vi "Write Waveform Type.vi"(8 "error in":errorcluster, 10 "Waveform Type":T1, 11 "Function Generator in":refnum<class "Function Generator.lvclass">) -> (0 "error out":errorcluster, 3 "Function Generator out":refnum<class "Function Generator.lvclass">)   [LabVIEW 2018, in "Function Generator.lvlib" / "Function Generator.lvclass"]
uses:
  Function Generator.lvclass
  Custom Controls/Waveform Type.ctl
  Function Generator.lvclass/Function Generator.ctl
  Function Generator.lvlib
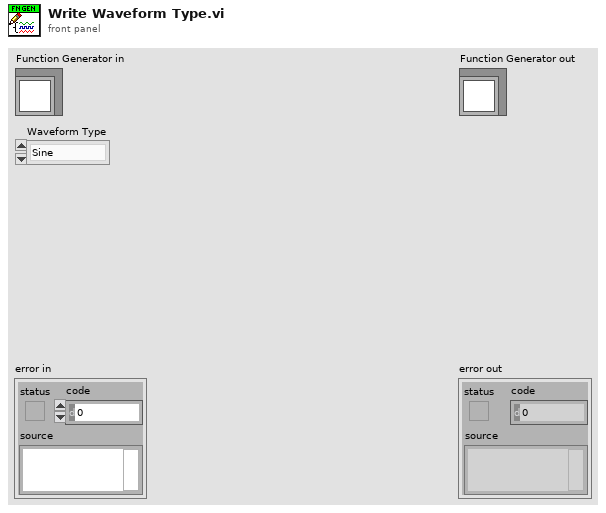
[diagram p1: front panel]
types:
  T1 = typedef "Function Generator.lvlib/Waveform Type.ctl" = enum16{"Sine", "Square", "Triangle", "Sawtooth", "DC"}
  T2 = typedef "Function Generator.lvlib/Channel Settings.ctl" = cluster{"Waveform Type":T1, "Amplitude Pk-Pk(V)":dbl, "Duty Cycle (%)":dbl, "Frequency (Hz)":dbl, "DC offset":dbl, "Output":bool}
  T3 = typedef "Function Generator.lvlib/Channel.ctl" = enum16{"Channel 1", "Channel 2", "Channel 3", "Channel 4"}
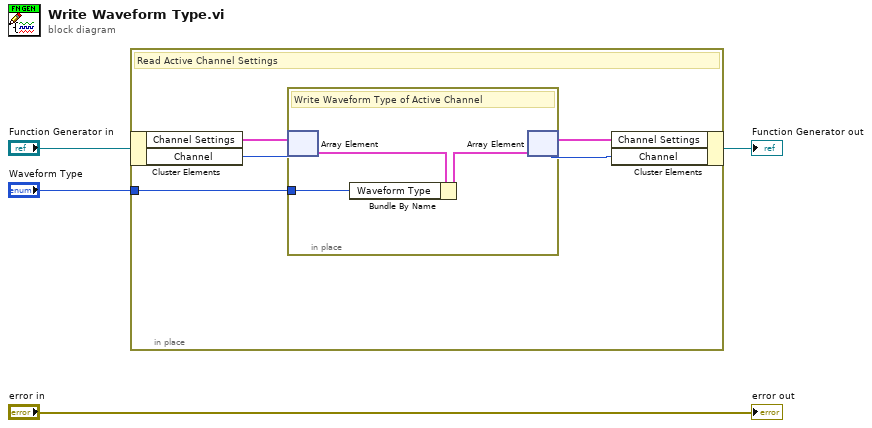
[diagram p0: block diagram]
diagram:
  n1 = in-place {
    in-place-border: "Waveform Type" -> [w5]
    # "Read Active Channel Settings"
    n2 = in-place-cluster #1("Function Generator in") -> ("Channel Settings"=w9:T2[], "Channel"=w8:T3)
    n3 = in-place {
      in-place-border: w5 -> [w10]
      # "Write Waveform Type of Active Channel"
      n4 = in-place-array #2(w9, w8) -> (w12:T2)
      n5 = Bundle By Name(cluster=w12, "Waveform Type"=w10) -> (w11:T2)
      n6 = in-place-array #2(w11) -> (w7:T2[], w6:i32)
    }
    n7 = in-place-cluster #1("Channel Settings"=w7, "Channel"=w6) -> (→"Function Generator out":refnum<class "Function Generator.lvclass">)
  }
  "error out" <- "error in"
